vi "getHexRotMat.vi"(8 "error in (no error)":errorcluster, 10 "Rotation Angle in Deg":dbl, 11 "CamRot in":refnum<class "CamRot.lvclass">) -> (0 "error out":errorcluster, 2 "Rotation Matrix":dbl[][](array[numeric]), 3 "CamRot out":refnum<class "CamRot.lvclass">)   [LabVIEW 2016, in "OfcFunc.lvlib" / "CamRot.lvclass"]
doc: "Get the hexapod rotation matrix."
uses:
  CamRot.lvclass
  MatOper/MatOper.lvclass
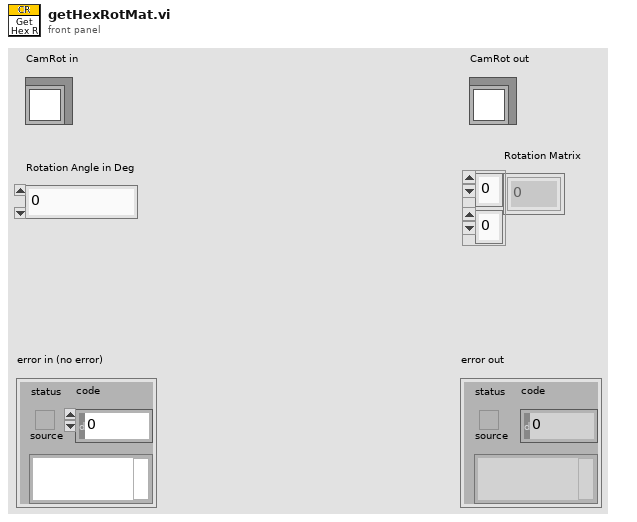
[diagram p1: front panel]
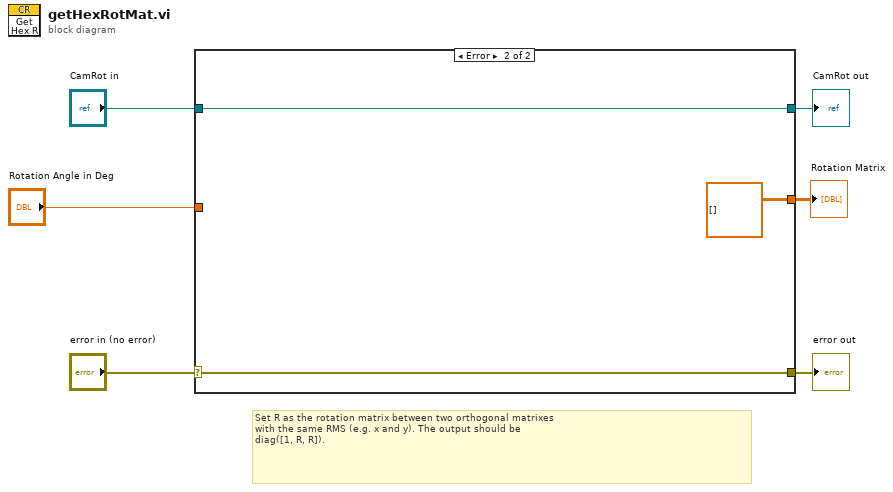
[diagram p0: block diagram]
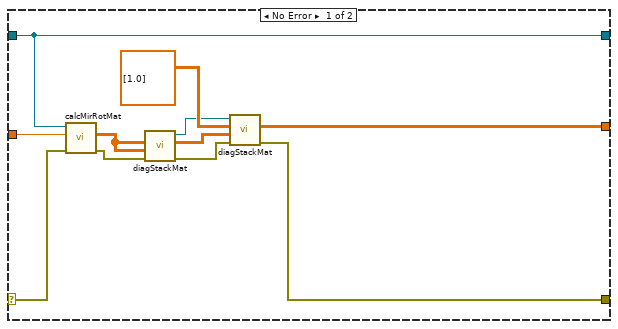
[diagram p2: hidden frame]
diagram:
  # "Set R as the rotation matrix between two orthogonal matrixes\nwith the same RMS (e.g. x and y). The output should be\ndiag([1, R, R])."
  n1 = case shown="Error" "error in (no error)" {
    selector: "error in (no error)" -> [w11 w20]
    tunnel: [w8 w20] -> w5
    tunnel: [w17 w19] -> w3
    tunnel: "CamRot in" -> [w17 w19]
    tunnel: "Rotation Angle in Deg" -> [w16 _]
    tunnel: [w12 dbl[][] [] ("Diag Stack Matrix")] -> w1
    frame No Error {
      n2 = call "calcMirRotMat.vi"("error in (no error)"=w11, "Rotation Angle in Deg"=w16, "CamRot in"=w17) -> ("error out"=w10:errorcluster, "Rotation Matrix"=w15:dbl[][])  [unwired: 6 in, 1 out]
      n3 = call "diagStackMat.vi"("error in (no error)"=w10, "A1"=w15, "A0"=w15) -> ("error out"=w9:errorcluster, "Diag Stack Matrix"=w13:dbl[][], "MatOper out"=w7:refnum<class "MatOper.lvclass">)  [unwired: 6 in]
      n4 = call "diagStackMat.vi"("error in (no error)"=w9, "A1"=w13, "A0"=dbl[][] [[1.0]], "MatOper in"=w7) -> ("error out"=w8:errorcluster, "Diag Stack Matrix"=w12:dbl[][])  [unwired: 5 in, 1 out]
    }
    frame Error {
    }
  }
  "error out" <- w5
  "CamRot out" <- w3
  "Rotation Matrix" <- w1
